vi "test.vi"() -> ()   [LabVIEW 2009]
panel:
  in  "stop":bool
  out "Loop Counter":u64
  out "Last Count Before Reset":u64
  in  "Add":bool
  in  "Reset":bool
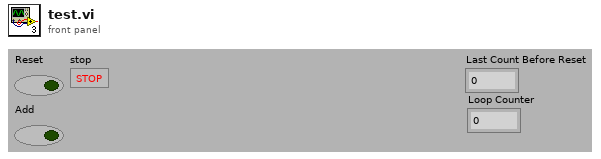
[diagram p1: front panel]
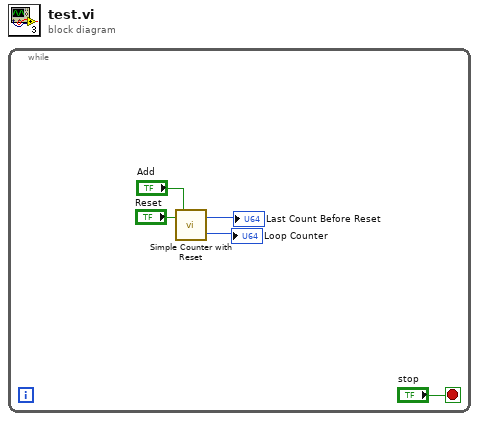
[diagram p0: block diagram]
diagram:
  n1 = while {
    stop <- "stop" stop-if-true
    n2 = call "Simple Counter with Reset.vi"("Add"="Add", "Reset"="Reset") -> ("Loop Counter"=→"Loop Counter":u64, "Last Count Before Reset"=→"Last Count Before Reset":u64)
  }
